vi "EnteringState.vi"(1 "IFw session":refnum<class "niInstr FIFO Register Bus v1 Host.lvclass">, 2 "FPGA Ref":refnum<k20>, 5 "SM inputs":T1, 9 "EnteringState":T2, 11 "error in (no error)":errorcluster) -> (15 "error out":errorcluster)   [LabVIEW 2017, in "AppStateMachine runtime.lvclass"]
uses:
  AppStateMachine runtime.lvclass
  State.ctl
  <instrlib>/_niInstr/FIFO Register Bus/v1/Host/niInstr FIFO Register Bus v1 Host.lvclass
  parameter user data.ctl
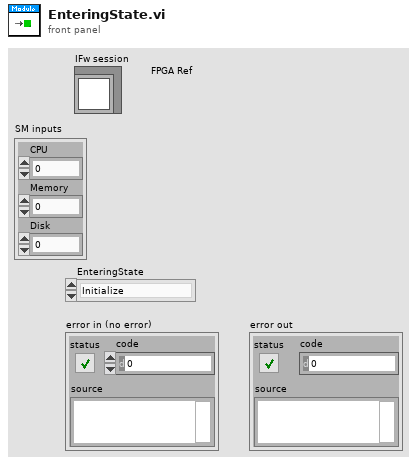
[diagram p1: front panel]
types:
  T1 = typedef "AppStateMachine runtime.lvclass/parameter user data.ctl" = cluster{"CPU":dbl, "Memory":dbl, "Disk":dbl}
  T2 = typedef "AppStateMachine runtime.lvclass/State.ctl" = enum16{"Initialize", "Idle", "Starting", "Running", "Stopping"}
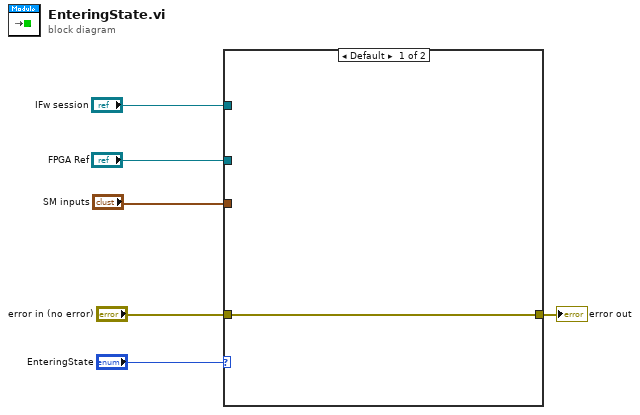
[diagram p0: block diagram]
diagram:
  n1 = case shown="Default" "EnteringState" {
    tunnel: "error in (no error)" -> [w7 w8]
    tunnel: [w7 w8] -> w6
    tunnel: "SM inputs" -> [_ _]
    tunnel: "IFw session" -> [_ _]
    tunnel: "FPGA Ref" -> [_ _]
    frame Default {
    }
    frame "Idle" {
    }
  }
  "error out" <- w6
